vi "clearpath_initialize_dataqueue.vi"(1 "Cluster":cluster{u8[], "Length":i32, "Type":i32}, 2 "Queue Name":string) -> (0 "Data Queue":refnum<queue>)   [LabVIEW 2010]
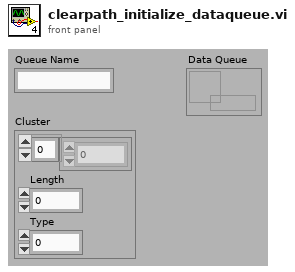
[diagram p1: front panel]
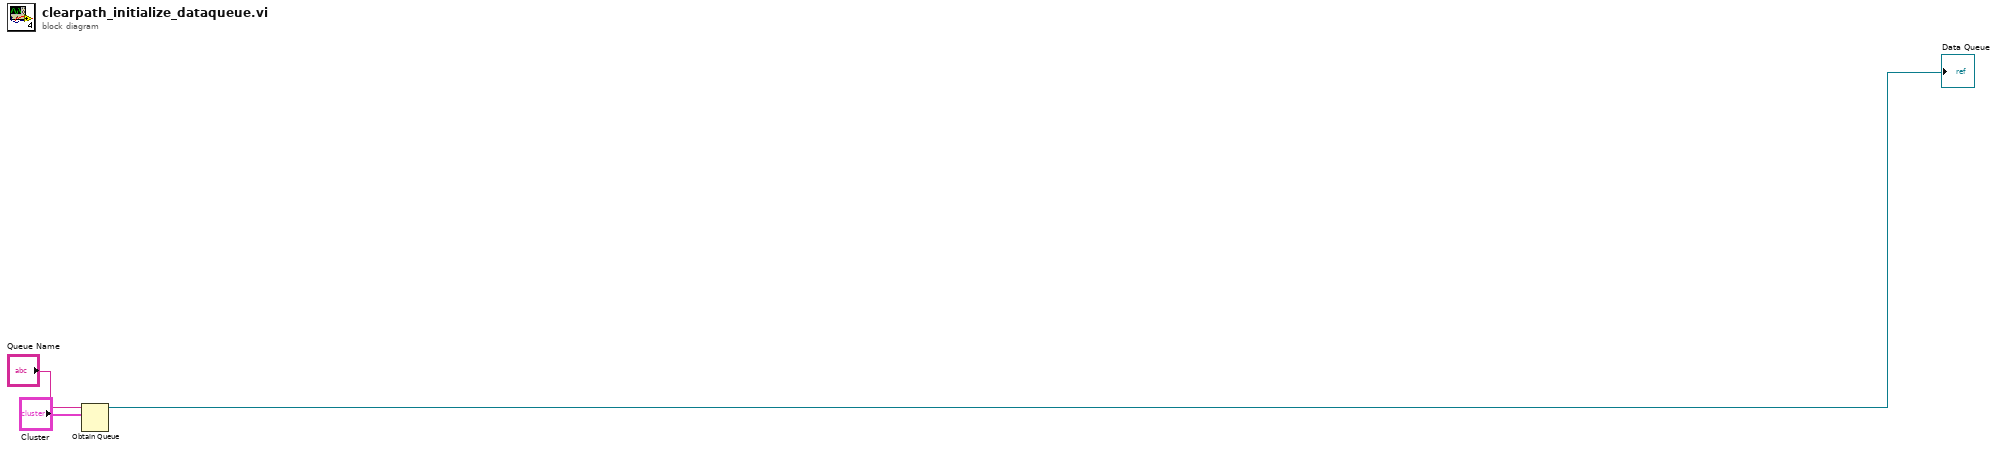
[diagram p0: block diagram]
diagram:
  n1 = Obtain Queue(name (unnamed)="Queue Name", element data type="Cluster") -> (queue out=→"Data Queue":refnum<queue>)  [unwired: 3 in, 2 out]
